vi "Elliptic Order Estimation.vi"(7 "filter type":T4, 8 "error in (no error)":errorcluster, 9 "ripple specs":T1={"passband"=0.1, "stopband"=60.0, "dB/linear? (T: dB)"=TRUE}, 10 "freq specs":T2={"lower pass freq"=0.2, "lower stop freq"=0.3, "higher pass freq"=0.0, "higher stop freq"=0.0}, 11 "sampling freq: fs":dbl=1.0 format="%.2f") -> (0 "error out":errorcluster, 1 "low cutoff freq":dbl, 2 "high cutoff freq":dbl, 3 "estimated order":i32, 4 "ripples [dB]":T3={"passband ripple"=1.0, "stopband atten"=60.0} {"stopband atten" format="%.2f"; "passband ripple" format="%.2f"})   [LabVIEW 2017, in "NI_AAL_Filter.lvlib"]
doc: "Estimates the Elliptic filter order."
uses:
  <vilib>/Analysis/NI_AAL_Filter.lvlib
  <vilib>/Analysis/3filter.llb/Filter Passband Type.ctl
  <vilib>/Analysis/3filter.llb/Filter Frequence Specification (Design).ctl
  <vilib>/Analysis/3filter.llb/Filter Ripple Specification (Design).ctl
  <vilib>/Analysis/NI_AALBase.lvlib
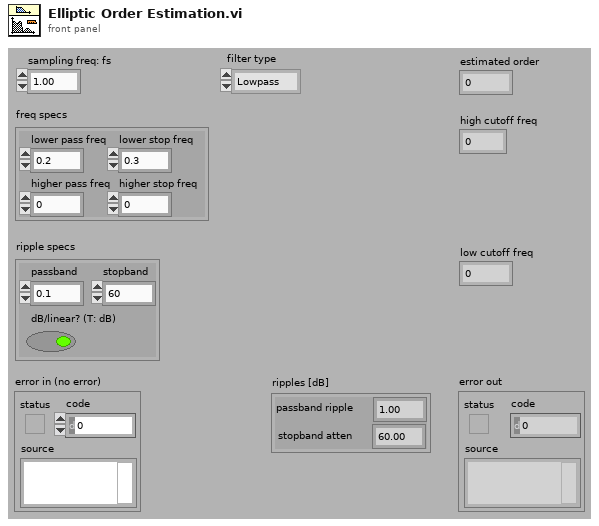
[diagram p1: front panel]
types:
  T1 = typedef "NI_AAL_Filter.lvlib/Filter Ripple Specification (Design).ctl" = cluster{"passband":dbl, "stopband":dbl, "dB/linear? (T: dB)":bool}
  T2 = typedef "NI_AAL_Filter.lvlib/Filter Frequence Specification (Design).ctl" = cluster{"lower pass freq":dbl, "lower stop freq":dbl, "higher pass freq":dbl, "higher stop freq":dbl}
  T3 = cluster{"passband ripple":dbl, "stopband atten":dbl}
  T4 = typedef "NI_AALBase.lvlib/Filter Passband Type.ctl" = enum32{"Lowpass", "Highpass", "Bandpass", "Bandstop"}
  T5 = enum16{"Butterworth", "Chebyshev", "Inverse Chebyshev", "Elliptic", "Bessel"}
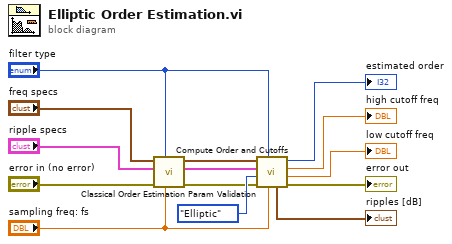
[diagram p0: block diagram]
diagram:
  n1 = call <vilib>:"Classical Order Estimation Param Validation.vi"("fs [Hz]"="sampling freq: fs", "filter type"="filter type", "error in (no error)"="error in (no error)", "ripple specs"="ripple specs", "freq specs [Hz]"="freq specs") -> ("error out"=w9:errorcluster, "dup ripple specs"=w7:T1, "dup freq specs [Hz]"=w8:T2)  [unwired: 1 in, 3 out]
  n2 = call <vilib>:"Compute Order and Cutoffs.vi"("fs [Hz]"="sampling freq: fs", "filter type"="filter type", "error in (no error)"=w9, "design method"=T5."Elliptic", "ripple specs"=w7, "freq specs [Hz]"=w8) -> ("error out"=→"error out":errorcluster, "low cutoff freq: fl"=→"low cutoff freq":dbl, "high cutoff freq: fh"=→"high cutoff freq":dbl, "n"=→"estimated order":i32, "ripples [dB]"=→"ripples [dB]":T3)  [unwired: 1 out]
